vi "Range Changer.vi"(11 "POV":i16) -> (3 "RPM":dbl format="%#_13g")   [LabVIEW 2016]
panel:
  in  "POV L RPM":dbl format="%#_13g"
  in  "POV B RPM":dbl format="%#_13g"
  in  "POV R RPM":dbl format="%#_13g"
  in  "POV F RPM":dbl format="%#_13g"
  in  "POV Left":i32=103
  in  "POV Back":i32
  in  "POV Right":i32=-43
  in  "POV Forward":i32=10
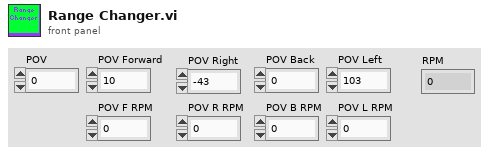
[diagram p1: front panel]
types:
  T1 = typedef "WPI_ServoDeviceRef.ctl" = cluster{"DeviceStatus":errorcluster, "PWM Channel":T2, "DeadBand":T3}
  T2 = typedef "FPGA_DIOPWMChannel.ctl" = enum8{"PWM 0", "PWM 1", "PWM 2", "PWM 3", "PWM 4", "PWM 5", "PWM 6", "PWM 7", "PWM 8", "PWM 9", "PWM MXP 0", "PWM MXP 1", "PWM MXP 2", "PWM MXP 3", "PWM MXP 4", "PWM MXP 5", "PWM MXP 6", "PWM MXP 7", "PWM MXP 8", "PWM MXP 9", "Invalid"}
  T3 = typedef "WPI_PWMDeadband.ctl" = cluster{"Name":string, "maxPositivePwm":i32, "minPositivePwm":i32, "centerPwm":i32, "maxNegativePwm":i32, "minNegativePwm":i32, "angularRange":u16}
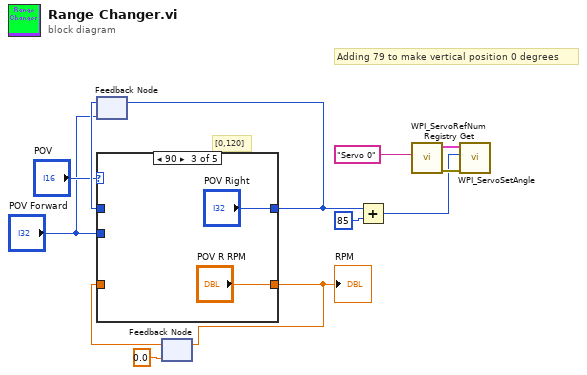
[diagram p0: block diagram]
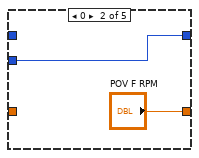
[diagram p3: hidden frame]
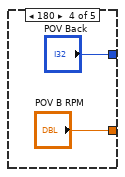
[diagram p4: hidden frame]
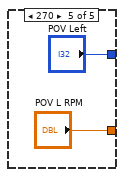
[diagram p5: hidden frame]
diagram:
  # "Adding 79 to make vertical position 0 degrees"
  # "[0,120]"
  n1 = feedback #1("POV Forward") -> (w10:i32)
  n2 = feedback #2(0.0 ("POV B RPM")) -> (w2:dbl)
  n3 = case shown="90" "POV" {
    tunnel: [w14 w15 "POV Right" "POV Back" "POV Left"] -> w8
    tunnel: w10 -> [w14 _ _ _ _]
    tunnel: [w13 "POV F RPM" "POV R RPM" "POV B RPM" "POV L RPM"] -> w4
    tunnel: w2 -> [w13 _ _ _ _]
    tunnel: "POV Forward" -> [_ w15 _ _ _]
    frame -1, Default {
    }
    frame 0 {
    }
    frame 90 {
    }
    frame 180 {
    }
    frame 270 {
    }
  }
  "RPM" <- w4
  n4 = feedback-in #1(w8) -> ()
  n5 = feedback-in #2(w4) -> ()
  n6 = Add(x=w8, y=85) -> (x+y=w6:i32)
  n7 = call <vilib>:"WPI_ServoRefNum Registry Get.vi"("refnum name"="Servo 0") -> ("error out"=w12:errorcluster, "ServoDeviceRef"=w11:T1)  [unwired: 9 in]
  n8 = call <vilib>:"WPI_ServoSetAngle.vi"("error in (no error)"=w12, "Angle"=w6, "ServoDeviceRef"=w11) -> ()  [unwired: 7 in, 2 out]
